vi "main(komplett).vi"() -> ()   [LabVIEW 2018]
doc: "MQTT Test using ThingSpeak channel 656489 (Test myRIO_rg)\n\nTreiber von cowen71, siehe\nC:\\Users\\Götting\\Documents\\LabVIEW Projekte\\mqtt-LabVIEW bzw. GitHub\n\nÄnderungen:\nkein Ping\nParameter (alle API Keys) für ThingSpeak Broker ok"
uses:
  src/class/mqtt/mqttTypedef/mqttSubscribeCluster.ctl
  src/class/mqtt/mqttTypedef/mqttQOSlevel.ctl
  src/class/mqtt/mqttTypedef/mqttConnectionStatus.ctl
  src/class/mqtt/mqttTXqueue/mqttTXdataQueueFunction.ctl
  src/class/mqtt/mqttConfigFunction.ctl
  src/class/mqtt/mqttTXqueue/mqttRXsubscriptionEventFunction.ctl
  src/class/mqtt/mqttTypedef/mqttBroker.ctl
  src/class/mqtt/mqttTypedef/mqttConnectionFlags.ctl
  src/class/mqtt/mqttTypedef/mqttWillInformation.ctl
  src/class/mqtt/mqttTypedef/mqttConnectionMeta.ctl
  src/class/mqtt/mqtt.lvclass
panel:
  out "Connects":i32
  out "messageID":u16
  out "RX Value":string
  out "RX Topic":string
  in  "disconnect":bool
  out "sessionPresent":bool
  out "Connect Status":T1
  in  "connect":bool
  in  "subscriptionInfo":T2[](array[typedef])=[{"Topic"="channels/656489/subscribe/fields/field1/RVIIFSV5FO3T3HVM", "QoS"=enum."At most once"}]
  out "subscribeMessageID":u16 format="%02x"
  out "Success":bool
  out "valueSent":string="14:19:17.238_"
  out "publishMessageID":u16 format="%02x"
  in  "value":string="field1=16"
  in  "topic":string="channels/656489/publish/8Q3U783L32ZXTE0U"
  in  "quit":bool
  in  "subscribe":bool
  in  "publish":bool
  out "error out":errorcluster
  # "MQTT Publish/Subscribe Client"
  # "Testprogramm/Demo mit Brokern:\nMosquitto/MacOS\nMosquitto/FabLab\nThingSpeak"
  # "Mosquitto/MacOS (139.13.78.42?): topic/state\nMosquitto/FabLab (139.13.82.5399: IOBroker/javascript/0/scriptEnabled/Honig/gewicht \nThingSpeak (mqtt.thingspeak.com): channels/656489/publish/8Q3U783L32ZXTE0U,\n   channels/656489/subscribe/fields/field1/RVIIFSV5FO3T3HVM"
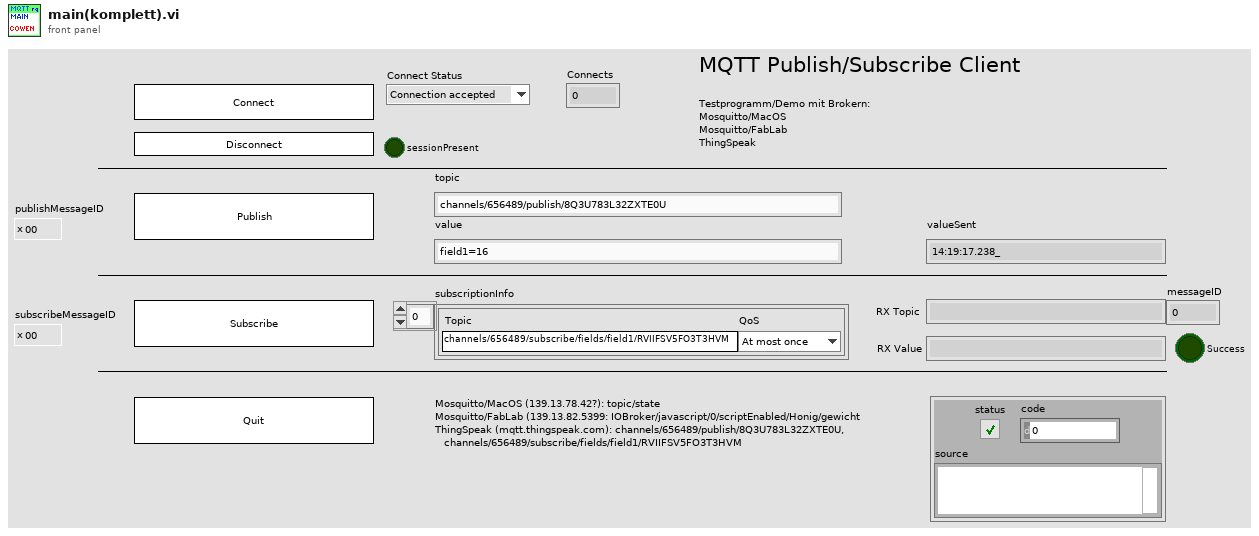
[diagram p1: front panel]
types:
  T1 = typedef "mqttConnectionStatus.ctl" = enum16{"Connection accepted", "Connection refused: unacceptable protocol version", "Connection refused: identifier rejected", "Connection refused: Server unavailable", "Connection refused: bad user name or password", "Connection refused: not authorized"}
  T2 = typedef "mqttSubscribeCluster.ctl" = cluster{"Topic":string, "QoS":T3}
  T3 = typedef "mqttQOSlevel.ctl" = enum8{"At most once", "At least once", "Exactly once", "Reserved"}
  T4 = typedef "mqttRXsubscriptionEventFunction.ctl" = enum16{"init", "deinit", "getEventRef", "event"}
  T5 = typedef "mqtt.lvclass/mqttConfigFunction.ctl" = enum16{"init", "deinit", "set", "get"}
  T6 = typedef "mqttTXdataQueueFunction.ctl" = enum16{"init", "deinit", "getQueue", "enqueue"}
  T7 = typedef "mqttBroker.ctl" = cluster{"address":string, "port":u16, "connTimeout":i32, "writeTimeout":i32, "readTimeout":i32, "subTimeout":i32}
  T8 = typedef "mqttConnectionFlags.ctl" = cluster{"reserved":bool, "clean session":bool, "will flag":bool, "willQOS":enum8{"At most once", "At least once", "Exactly once", "Reserved"}, "will retain":bool, "password":bool, "user name":bool}
  T9 = typedef "mqttWillInformation.ctl" = cluster{"User Name":string, "Password":string}
  T10 = cluster{"ClientID":string, "Broker":T7, "Flags":T8, "User Info":T9}
  T11 = enum8{"Enabled", "Disabled", "Disabled and Grayed Out"}
  T12 = typedef "mqttConnectionMeta.ctl" = cluster{"retain":bool, "duplicate":bool, "qos":T3}
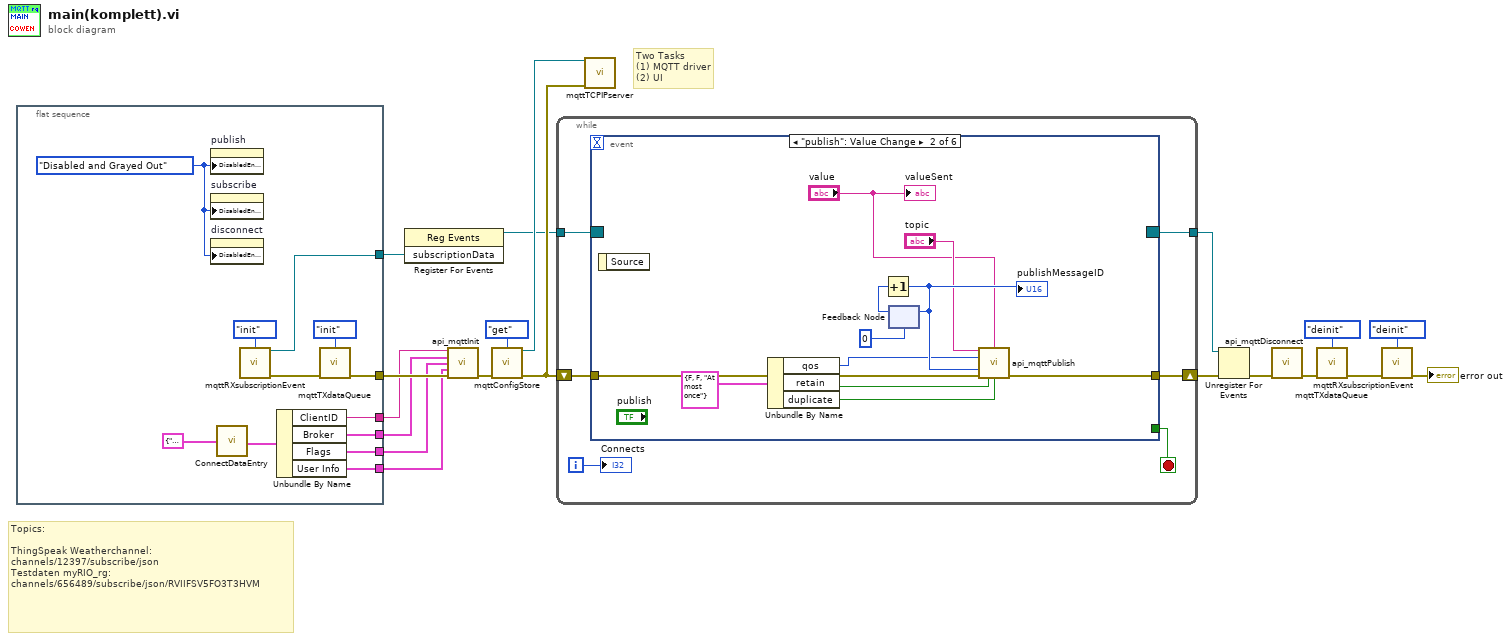
[diagram p0: block diagram]
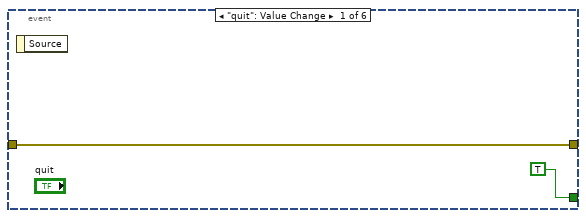
[diagram p2: hidden frame]
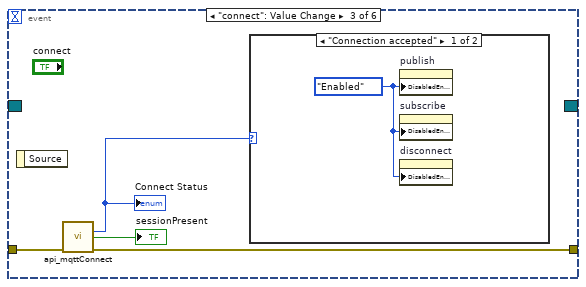
[diagram p3: hidden frame]
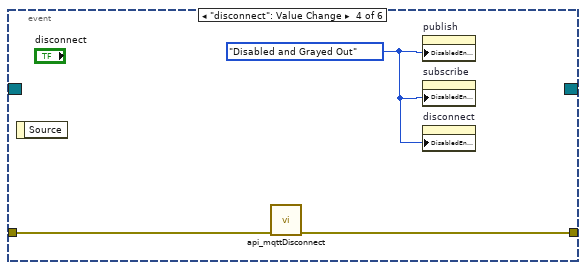
[diagram p5: hidden frame]
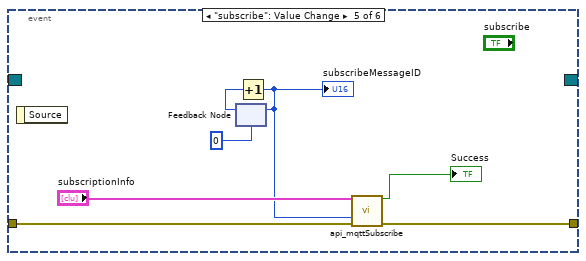
[diagram p6: hidden frame]
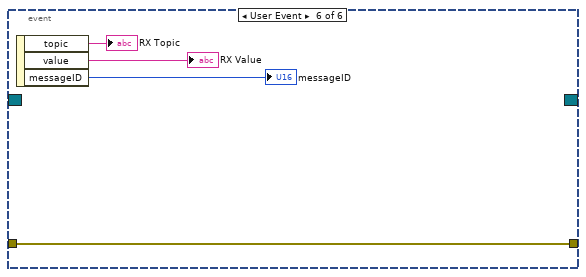
[diagram p7: hidden frame]
diagram:
  # "Two Tasks\n(1) MQTT driver\n(2) UI"
  # "Topics:\n\nThingSpeak Weatherchannel:\nchannels/12397/subscribe/json\nTestdaten myRIO_rg:\nchannels/656489/subscribe/json/RVIIFSV5FO3T3HVM"
  n1 = flat-sequence {
    tunnel: [w30] -> w18
    tunnel: [w27] -> w12
    tunnel: [w25] -> w4
    tunnel: [w24] -> w3
    tunnel: [w23] -> w2
    tunnel: [w22] -> w1
    frame #0 {
      w26 = T11."Disabled and Grayed Out" ("Disabled")
      n2 = property on="publish" class="Bool"("DisabledEnum"=w26) -> ()  [unwired: 2 in, 2 out]
      n3 = property on="subscribe" class="Bool"("DisabledEnum"=w26) -> ()  [unwired: 2 in, 2 out]
      n4 = property on="disconnect" class="Bool"("DisabledEnum"=w26) -> ()  [unwired: 2 in, 2 out]
      n5 = call "ConnectDataEntry.vi"("MQTT Connect Data in"=T10 {"ClientID"="44be5e2ab7441ebaed34d7fa45d5e0", "Broker"={"address"="mqtt.thingspeak.com", "port"=1883, "connTimeout"=2000, "writeTimeout"=2000, "readTimeout"=2000, "subTimeout"=30000}, "Flags"={"reserved"=FALSE, "clean session"=TRUE, "will flag"=FALSE, "willQOS"=enum."At most once", "will retain"=FALSE, "password"=TRUE, "user name"=TRUE}, "User Info"={"User Name"="rgoetting", "Password"="2V41PDRHCBV3T4MR"}}) -> ("MQTT Connect Data out"=w21:T10)  [unwired: 4 in]
      n6 = call "mqttRXsubscriptionEvent.vi"("function"=mqttRXsubscriptionEventFunction."init") -> ("subscriptionData"=w27:refnum<user-event>, "error out"=w29:errorcluster)  [unwired: 13 in]
      n7 = Unbundle By Name(w21) -> ("ClientID"=w25:string, "Broker"=w24:T7, "Flags"=w23:T8, "User Info"=w22:T9)
      n8 = call "mqttTXdataQueue.vi"("function"=mqttTXdataQueueFunction."init", "error in (no error)"=w29) -> ("error out"=w30:errorcluster)  [unwired: 12 in, 1 out]
    }
  }
  n9 = register-events(w12) -> (reference out=w11:refnum<event-registration>)  [unwired: 2 in, 1 out]
  n10 = call "api_mqttInit.vi"("client"=w4, "broker"=w3, "connFlags"=w2, "User Info"=w1, "error in (no error)"=w18) -> ("error out"=w16:errorcluster)  [unwired: 10 in]
  n11 = call "mqttConfigStore.vi"("function"=mqttConfigFunction."get", "error in (no error)"=w16) -> ("mqtt.lvclass out"=w15:refnum<class "mqtt.lvclass">, "error out"=w14:errorcluster)  [unwired: 12 in]
  n12 = while {
    shift-right: [w37] -> w7
    shift-left: w14 -> [w36]
    tunnel: w11 -> [w34]
    tunnel: [w32] -> w5
    i -> [w33]
    stop <- w35 stop-if-true
    n13 = event shown="[1] \"publish\": Value Change" {
      selector: w34 -> [_ _ _ _ _ _]
      dyn-events: [_ _ _ _ _ _] -> w32
      timeout: _ -> [_ _ _ _ _ _]
      tunnel: [w38 w47 w53 w57 w61 w69] -> w37
      tunnel: w36 -> [w38 w48 w54 w58 w59 w69]
      tunnel: [TRUE _ _ _ _ _] -> w35
      event "quit": Value Change {
        n14 = event-data() -> ()  [unwired: 1 in, 1 out]
      }
      event "publish": Value Change {
        n15 = event-data() -> ()  [unwired: 1 in, 1 out]
        n16 = Unbundle By Name(T12 {"retain"=FALSE, "duplicate"=FALSE, "qos"=enum."At most once"} ("connMeta")) -> ("qos"=w42:T3, "retain"=w44:bool, "duplicate"=w40:bool)
        n17 = feedback #1(u16 0) -> (w49:u16)
        n18 = Increment(x=w49) -> (x+1=w46:u16)
        "publishMessageID" <- w46
        n19 = feedback-in #1(w46) -> ()
        n20 = call "api_mqttPublish.vi"("topic"="topic", "value"="value", "QoS (At most once)"=w42, "messageID"=w46, "error in (no error)"=w48, "retain(F)"=w44, "duplicate(F)"=w40) -> ("error out"=w47:errorcluster)  [unwired: 7 in, 1 out]
        "valueSent" <- "value"
      }
      event "connect": Value Change {
        n21 = event-data() -> ()  [unwired: 1 in, 1 out]
        n22 = call "api_mqttConnect.vi"("error in (no error)"=w54) -> ("connStatus"=w51:T1, "sessionPresent"=→"sessionPresent":bool, "error out"=w53:errorcluster)  [unwired: 11 in, 1 out]
        "Connect Status" <- w51
        n23 = case shown="\"Connection accepted\"" w51 {
          frame "Connection accepted" {
            w55 = T11."Enabled" ("Disabled")
            n24 = property on="publish" class="Bool"("DisabledEnum"=w55) -> ()  [unwired: 2 in, 2 out]
            n25 = property on="subscribe" class="Bool"("DisabledEnum"=w55) -> ()  [unwired: 2 in, 2 out]
            n26 = property on="disconnect" class="Bool"("DisabledEnum"=w55) -> ()  [unwired: 2 in, 2 out]
          }
          frame Default {
          }
        }
      }
      event "disconnect": Value Change {
        w56 = T11."Disabled and Grayed Out" ("Disabled")
        n27 = event-data() -> ()  [unwired: 1 in, 1 out]
        n28 = call "api_mqttDisconnect.vi"("error in (no error)"=w58) -> ("error out"=w57:errorcluster)  [unwired: 13 in, 1 out]
        n29 = property on="publish" class="Bool"("DisabledEnum"=w56) -> ()  [unwired: 2 in, 2 out]
        n30 = property on="subscribe" class="Bool"("DisabledEnum"=w56) -> ()  [unwired: 2 in, 2 out]
        n31 = property on="disconnect" class="Bool"("DisabledEnum"=w56) -> ()  [unwired: 2 in, 2 out]
      }
      event "subscribe": Value Change {
        n32 = event-data() -> ()  [unwired: 1 in, 1 out]
        n33 = feedback #2(u16 0) -> (w64:u16)
        n34 = Increment(x=w64) -> (x+1=w60:u16)
        "subscribeMessageID" <- w60
        n35 = feedback-in #2(w60) -> ()
        n36 = call "api_mqttSubscribe.vi"("subscriptionInfo"="subscriptionInfo", "messageID"=w60, "error in (no error)"=w59) -> ("success"=→"Success":bool, "error out"=w61:errorcluster)  [unwired: 11 in]
      }
      event User Event {
        n37 = event-data() -> ("topic"=→"RX Topic":string, "value"=→"RX Value":string, "messageID"=→"messageID":u16)  [unwired: 1 in]
      }
    }
    "Connects" <- w33
  }
  n38 = call "mqttTCPIPserver.vi"("mqtt.lvclass"=w15, "error in (no error)"=w14) -> ()  [unwired: 12 in, 2 out]
  n39 = Unregister For Events(event registration refnum=w5, error in=w7) -> (error out=w6:errorcluster)
  n40 = call "api_mqttDisconnect.vi"("error in (no error)"=w6) -> ("error out"=w13:errorcluster)  [unwired: 13 in, 1 out]
  n41 = call "mqttTXdataQueue.vi"("function"=mqttTXdataQueueFunction."deinit", "error in (no error)"=w13) -> ("error out"=w9:errorcluster)  [unwired: 12 in, 1 out]
  n42 = call "mqttRXsubscriptionEvent.vi"("function"=mqttRXsubscriptionEventFunction."deinit", "error in (no error)"=w9) -> ("error out"=→"error out":errorcluster)  [unwired: 12 in, 1 out]
